vi "example_2_2_c.vi"() -> ()   [LabVIEW 2018]
panel:
  out "Numeric":dbl format="%.2f"
  in  "Knob":dbl(knob) scale=0.0..10.0 scale format="%.1f"
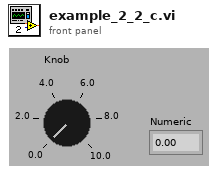
[diagram p1: front panel]
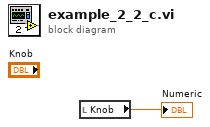
[diagram p0: block diagram]
diagram:
  n1 = local read "Knob"() -> (→"Numeric":dbl)
